vi "Read Time Stamp.vi"(8 "error in":errorcluster, 11 "Has Timestamp in":refnum<class "Has Time Stamp.lvclass">) -> (0 "error out":errorcluster, 1 "user tag":i32, 2 "time stamp":timestamp, 3 "Has Timestamp out":refnum<class "Has Time Stamp.lvclass">)   [LabVIEW 2020, in "PV Access.lvlib" / "PV Data.lvlib" / "Has Time Stamp.lvclass"]
uses:
  Has Time Stamp.lvclass
  PV Data.lvlib
  EPICS Time Stamp.ctl
  3a2aeaae-d079-45d7-aa80-7f158ca5949c.vi
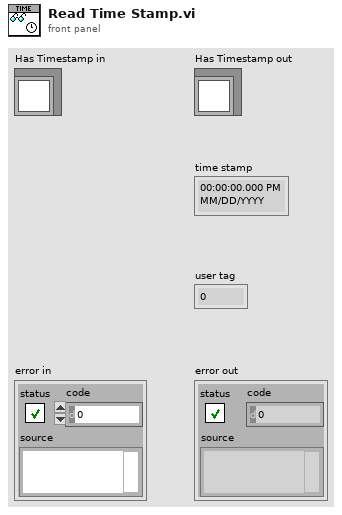
[diagram p1: front panel]
types:
  T1 = typedef "PV Access.lvlib/PV Data.lvlib/EPICS Time Stamp.ctl" = cluster{"secondsPastEpoch":i64, "nanoseconds":i32, "userTag":i32}
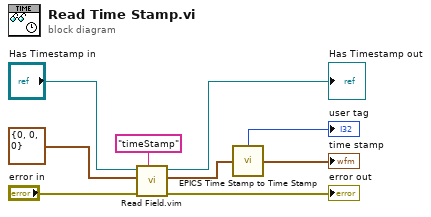
[diagram p0: block diagram]
diagram:
  n1 = call "Read Field.vim"("field"="timeStamp" ("element name"), "error in"="error in", "default value"=T1 {"secondsPastEpoch"=0, "nanoseconds"=0, "userTag"=0} ("timeStamp"), "Base Interface in"="Has Timestamp in") -> ("error out"=→"error out":errorcluster, "value"=w3:T1, "Base Interface out"=→"Has Timestamp out":refnum<class "Has Time Stamp.lvclass">)  [unwired: 5 in]
  n2 = call "EPICS Time Stamp to Time Stamp.vi"("EPICS time stamp"=w3) -> ("user tag"=→"user tag":i32, "time stamp"=→"time stamp":timestamp)
